vi "stop.vi"() -> ()   [LabVIEW 2016]
uses:
  <vilib>/NXT/Subs/LVHSConnector.ctl
  <vilib>/NXT/LegoClasses/BrickReference/BrickReference.lvclass
  <vilib>/NXT/Block Support/NXT_InputPort.ctl
  <vilib>/NXT/Block Support/NXT_OutputPort.ctl
  <vilib>/NXT/NXTIO Xnodes/NXTIONodeSubVIs/NXTStopMotors.vi
  <vilib>/NXT/NXTIO Xnodes/NXTIONodeSubVIs/NXTMoveMotors.vi
  <vilib>/NXT/NXTIO Xnodes/AddressXNode/NXTIOAddress.xnode
  <vilib>/NXT/NXTIO Xnodes/NXTIOXNode/NXTIO.xnode
panel:
  out "Distance (cm) 2":i16
  out "Degrees":sgl
  out "NXT/EV3 2":T1
  in  "NXT/EV3":T1
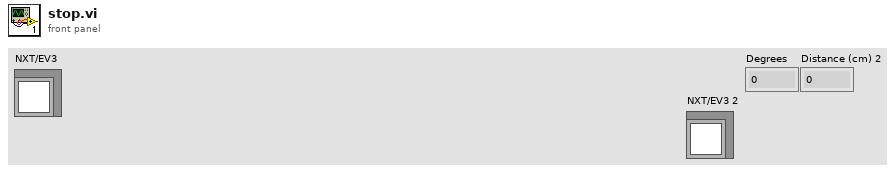
[diagram p1: front panel]
types:
  T1 = typedef "LVHSConnector.ctl" = refnum<class "BrickReference.lvclass">
  T2 = typedef "NXT_InputPort.ctl" = u32
  T3 = typedef "NXT_OutputPort.ctl" = u8
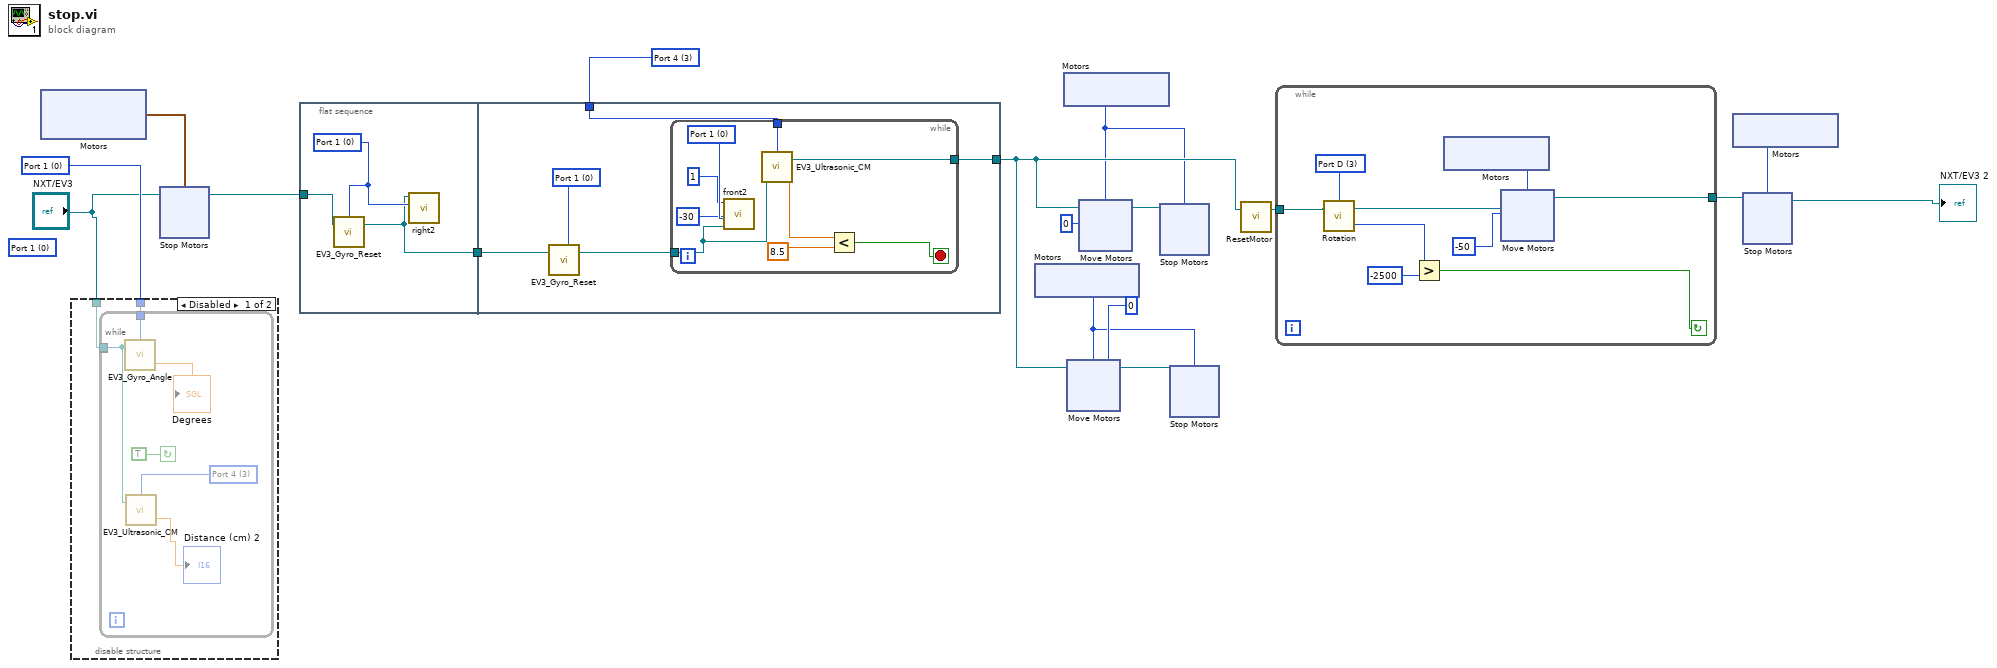
[diagram p0: block diagram]
diagram:
  (unwired) T2 0 items=["Port 1", "Port 2", "Port 3", "Port 4"] ("Port (Port 1)")
  w11 = T2 0 items=["Port 1", "Port 2", "Port 3", "Port 4"] ("Port (Port 1)")
  w10 = T2 3 items=["Port 1", "Port 2", "Port 3", "Port 4"] ("Port (Port 4)")
  n1 = xnode "Motors"() -> ("Motor"=w16:cluster{"Port":T3, "Port":T3})
  n2 = disable-structure shown="Disabled" {
    disable-tunnel: w11 -> [w19 _]
    disable-tunnel: "NXT/EV3" -> [w18 _]
    frame Disabled {
      n3 = while {
        tunnel: w19 -> [w25]
        tunnel: [w20] -> _
        tunnel: w18 -> [w20]
        stop <- TRUE continue-if-true
        w22 = T2 3 items=["Port 1", "Port 2", "Port 3", "Port 4"] ("Port (Port 4)")
        n4 = call <vilib>:"EV3_Gyro_Angle.vi"("NXT/EV3"=w20, "Port (Port 1)"=w25) -> ("Degrees"=→"Degrees":sgl)  [unwired: 1 in, 1 out]
        n5 = call <vilib>:"EV3_Ultrasonic_CM.vi"("NXT/EV3"=w20, "Port (Port 1)"=w22) -> ("Centimeters"=→"Distance (cm) 2":sgl)  [unwired: 1 in, 1 out]
      }
    }
    frame Enabled {
    }
  }
  n6 = xnode "Stop Motors"("Motors"=w16, "NXT/EV3"="NXT/EV3") -> ("NXT/EV3"=w17:T1)
  n7 = flat-sequence {
    tunnel: w17 -> [w28]
    tunnel: [w26] -> w1
    tunnel: w10 -> [w33]
    tunnel: [w30] -> w9
    tunnel: w1 -> [w29]
    frame #0 {
      w27 = T2 0 items=["Port 1", "Port 2", "Port 3", "Port 4"] ("Gyro Port")
      n8 = call <vilib>:"EV3_Gyro_Reset.vi"("NXT/EV3"=w28, "Port (Port 1)"=w27) -> ("NXT/EV3"=w26:T1)  [unwired: 2 in]
      n9 = call "right2.vi"("Gyro Port"=w27, "NXT/EV3"=w26) -> ()  [unwired: 9 in, 1 out]
    }
    frame #1 {
      w32 = T2 0 items=["Port 1", "Port 2", "Port 3", "Port 4"] ("Port (Port 1)")
      n10 = call <vilib>:"EV3_Gyro_Reset.vi"("NXT/EV3"=w29, "Port (Port 1)"=w32) -> ("NXT/EV3"=w31:T1)  [unwired: 2 in]
      n11 = while {
        tunnel: w33 -> [w42]
        tunnel: w31 -> [w37]
        tunnel: [w35] -> w30
        stop <- w41 stop-if-true
        w39 = T2 0 items=["Port 1", "Port 2", "Port 3", "Port 4"] ("Gyro Port")
        n12 = call "front2.vi"("NXT/EV3"=w37, "Gyro Port"=w39, "Motor speed"=-30, "Kp"=1) -> ()  [unwired: 8 in]
        n13 = call <vilib>:"EV3_Ultrasonic_CM.vi"("NXT/EV3"=w37, "Port (Port 1)"=w42) -> ("Centimeters"=w40:sgl, "NXT/EV3"=w35:T1)  [unwired: 1 in]
        n14 = Less?(x=w40, y=8.5) -> (x < y?=w41:bool)
      }
    }
  }
  n15 = xnode "Motors"() -> ("Motor"=w3:T3)
  n16 = xnode "Motors"() -> ("Motor"=w2:T3)
  n17 = xnode "Move Motors"("Power/Speed 1"=i8 0, "Motors"=w3, "NXT/EV3"=w9) -> ("NXT/EV3"=w4:T1)
  n18 = xnode "Move Motors"("Power/Speed 1"=i8 0, "Motors"=w2, "NXT/EV3"=w9) -> ("NXT/EV3"=w5:T1)
  n19 = xnode "Stop Motors"("Motors"=w2, "NXT/EV3"=w5) -> ()  [unwired: 1 out]
  n20 = xnode "Stop Motors"("Motors"=w3, "NXT/EV3"=w4) -> ()  [unwired: 1 out]
  n21 = call <vilib>:"ResetMotor.vi"("NXT/EV3"=w9) -> ("NXT/EV3"=w15:T1)  [unwired: 3 in]
  n22 = while {
    tunnel: w15 -> [w51]
    tunnel: [w43] -> w14
    stop <- w47 continue-if-true
    w50 = T3 3 items=["Port A", "Port B", "Port C", "Port D"] ("Port (Port A)")
    n23 = call <vilib>:"Rotation.vi"("NXT/EV3"=w51, "Port (Port A)"=w50) -> ("Angle of Rotation"=w49:i32, "NXT/EV3"=w45:T1)  [unwired: 1 in]
    n24 = Greater?(x=w49, y=-2500) -> (0:w47:bool)
    n25 = xnode "Motors"() -> ("Motor"=w46:T3)
    n26 = xnode "Move Motors"("Power/Speed 1"=i8 -50, "Motors"=w46, "NXT/EV3"=w45) -> ("NXT/EV3"=w43:T1)
  }
  n27 = xnode "Motors"() -> ("Motor"=w13:T3)
  n28 = xnode "Stop Motors"("Motors"=w13, "NXT/EV3"=w14) -> ("NXT/EV3"=→"NXT/EV3 2":T1)
